vi "TimeStamp to Cron Time.vi"(11 "Time Stamp":timestamp) -> (3 "Cron Time":T1)   [LabVIEW 2013, in "openCron.lvlib" / "Cron.lvclass"]
uses:
  Cron.lvclass
  CronTime -- cluster.ctl
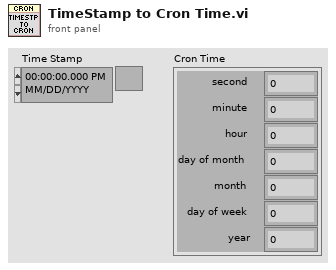
[diagram p1: front panel]
types:
  T1 = typedef "openCron.lvlib/Cron.lvclass/CronTime -- cluster.ctl" = cluster{"second":i32, "minute":i32, "hour":i32, "day of month":i32, "month":i32, "day of week":i32, "year":i32}
  T2 = typedef "LVDateTimeRec.ctl" = cluster{"fractional second":dbl, "second":i32, "minute":i32, "hour":i32, "day of month":i32, "month":i32, "year":i32, "day of week":i32, "day of year":i32, "DST":i32}
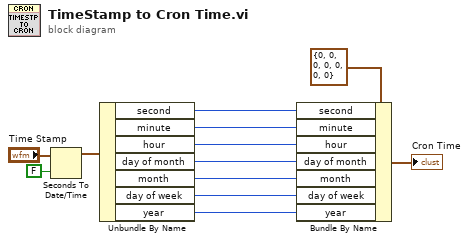
[diagram p0: block diagram]
diagram:
  n1 = Seconds To Date/Time(time stamp (now)="Time Stamp", to UTC (F)=FALSE) -> (date time rec=w2:T2)
  n2 = Unbundle By Name(w2) -> ("second"=w4:i32, "minute"=w5:i32, "hour"=w6:i32, "day of month"=w7:i32, "month"=w8:i32, "day of week"=w9:i32, "year"=w10:i32)
  n3 = Bundle By Name(cluster=T1 {"second"=0, "minute"=0, "hour"=0, "day of month"=0, "month"=0, "day of week"=0, "year"=0} ("Cron"), "second"=w4, "minute"=w5, "hour"=w6, "day of month"=w7, "month"=w8, "day of week"=w9, "year"=w10) -> (→"Cron Time":T1)
